vi "Sel Biometry State.vi"(8 "error in (no error)":errorcluster caption="错误输入（无错误）", 9 "condition":string, 11 "connection reference":T2) -> (0 "error out":errorcluster caption="错误输出", 2 "Biometry State":T1[](array[typedef]))   [LabVIEW 2015, in "Database Processing.lvlib"]
doc: "该模板用于创建子VI。"
uses:
  Database Processing.lvlib
  <vilib>/addons/database/Connection.llb/Conn ObjectReference.ctl
  Support/Table/Biometry State.ctl
  <vilib>/addons/database/_DB Variant To Data/Database Variant To Data.xnode
  <vilib>/addons/database/NI_Database_API.lvlib
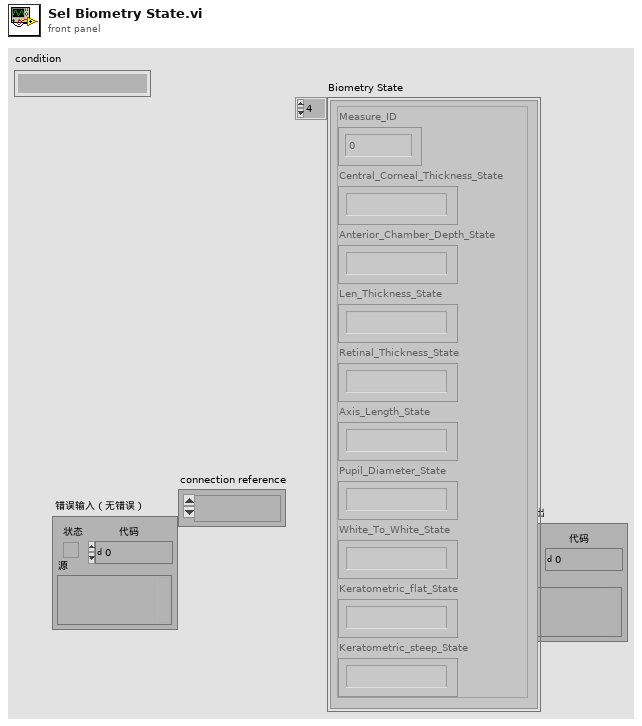
[diagram p1: front panel]
types:
  T1 = typedef "Database Processing.lvlib/Biometry State.ctl" = cluster{"Measure_ID":i64, "Central_Corneal_Thickness_State":string, "Anterior_Chamber_Depth_State":string, "Len_Thickness_State":string, "Retinal_Thickness_State":string, "Axis_Length_State":string, "Pupil_Diameter_State":string, "White_To_White_State":string, "Keratometric_flat_State":string, "Keratometric_steep_State":string}
  T2 = typedef "NI_Database_API.lvlib/Conn ObjectReference.ctl" = refnum<k1>
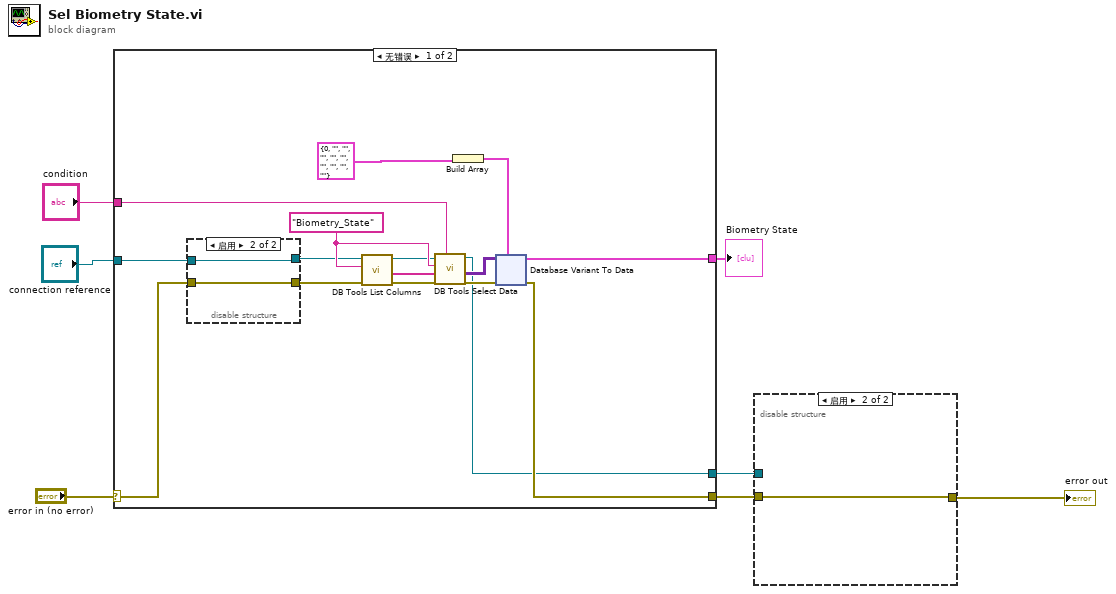
[diagram p0: block diagram]
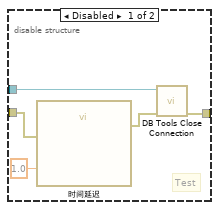
[diagram p2: hidden frame]
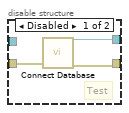
[diagram p3: hidden frame]
diagram:
  n1 = case shown="无错误" "error in (no error)" {
    selector: "error in (no error)" -> [w11 w350]
    tunnel: [w20 w350] -> w3
    tunnel: "connection reference" -> [w13 w349]
    tunnel: [w16 _] -> w1
    tunnel: "condition" -> [w15 _]
    tunnel: [w9 w349] -> w4
    frame No Error {
      w17 = "Biometry_State" ("table")
      n2 = disable-structure shown="启用" {
        disable-tunnel: [w26 w28] -> w14
        disable-tunnel: w13 -> [_ w28]
        disable-tunnel: w11 -> [w25 w27]
        disable-tunnel: [w24 w27] -> w12
        frame Disabled {
          # "Test"
          n3 = call "Connect Database.vi"("error in (no error)"=w25) -> ("error out"=w24:errorcluster, "connection reference"=w26:T2)  [unwired: 9 in]
        }
        frame Enabled {
        }
      }
      n4 = call <vilib>:"DB Tools List Columns.vi"("error in (no error)"=w12, "table"=w17, "connection reference"=w14) -> ("error out"=w19:errorcluster, "columns"=w18:string[], "connection reference out"=w10:T2)  [unwired: 1 in, 1 out]
      n5 = call <vilib>:"DB Tools Select Data.vi"("condition"=w15, "error in (no error)"=w19, "columns"=w18, "table"=w17, "connection reference"=w10) -> ("error out"=w23:errorcluster, "data"=w22:variant[][], "connection reference out"=w9:T2)  [unwired: 1 in]
      n6 = Build Array(T1 {"Measure_ID"=0, "Central_Corneal_Thickness_State"="", "Anterior_Chamber_Depth_State"="", "Len_Thickness_State"="", "Retinal_Thickness_State"="", "Axis_Length_State"="", "Pupil_Diameter_State"="", "White_To_White_State"="", "Keratometric_flat_State"="", "Keratometric_steep_State"=""} ("Biometry State")) -> (w21:T1[])
      n7 = xnode "Database Variant To Data"("database variant"=w22, "error in (no error)"=w23, "type"=w21) -> ("data"=w16:T1[], "error out"=w20:errorcluster)
    }
    frame Error {
    }
  }
  "Biometry State" <- w1
  n8 = disable-structure shown="启用" {
    disable-tunnel: w3 -> [w353 w356]
    disable-tunnel: [w355 w356] -> w2
    disable-tunnel: w4 -> [w354 _]
    frame Disabled {
      # "Test"
      n9 = call "时间延迟"("error in (no error)"=w353, "Delay Time (s)"=1.0) -> ("error out"=w352:errorcluster)  [unwired: 9 in]
      n10 = call <vilib>:"DB Tools Close Connection.vi"("error in (no error)"=w352, "connection reference"=w354) -> ("error out"=w355:errorcluster)  [unwired: 5 in]
    }
    frame Enabled {
    }
  }
  "error out" <- w2
